vi "vi_package_setup_coordinator.vi"(8 "error in (no error)":errorcluster, 9 "Set":bool=TRUE, 10 "value":string, 11 "name in":string) -> (0 "error out":errorcluster, 1 "Found":bool, 2 "replaced":bool, 3 "values":string)   [LabVIEW 2021]
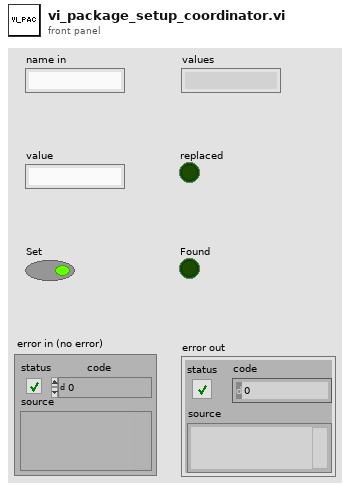
[diagram p1: front panel]
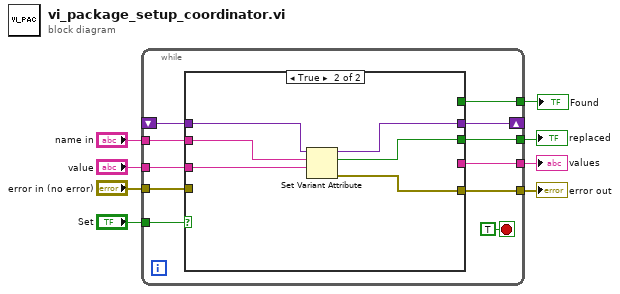
[diagram p0: block diagram]
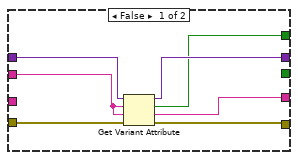
[diagram p2: hidden frame]
diagram:
  n1 = while {
    tunnel: "Set" -> [w19]
    tunnel: "name in" -> [w17]
    tunnel: "value" -> [w16]
    shift-right: [w15] -> _
    shift-left: _ -> [w14]
    tunnel: [w13] -> w5
    tunnel: [w12] -> w4
    tunnel: [w11] -> w3
    tunnel: [w10] -> w2
    tunnel: "error in (no error)" -> [w9]
    stop <- TRUE stop-if-true
    n2 = case shown="True" w19 {
      tunnel: w17 -> [w21 w32]
      tunnel: w16 -> [_ w31]
      tunnel: [w25 w30] -> w15
      tunnel: w14 -> [w26 w27]
      tunnel: [w24 w29] -> w13
      tunnel: [w20 _] -> w12
      tunnel: [_ w28] -> w11
      tunnel: [w23 _] -> w10
      tunnel: w9 -> [w22 _]
      frame False {
        n3 = Get Variant Attribute(Variant=w26, name=w21, default value (empty Variant)=w21, error in=w22) -> (duplicate Variant=w25:variant, found=w23:bool, value=w20:string, error out=w24:errorcluster)
      }
      frame True {
        n4 = Set Variant Attribute(Variant=w27, name=w32, value=w31) -> (Variant out=w30:variant, replaced=w28:bool, error out=w29:errorcluster)  [unwired: 1 in]
      }
    }
  }
  "error out" <- w5
  "values" <- w4
  "replaced" <- w3
  "Found" <- w2
